vi "ArduinoCommand.vi"(8 "entrée d'erreur (pas d'erreur)":errorcluster, 10 "buffer à écrire":string, 11 "Refnum VISA en entrée":refnum<visa-resource-name>) -> (0 "sortie d'erreur":errorcluster, 2 "read buffer":string, 3 "Refnum VISA en sortie":refnum<visa-resource-name>)   [LabVIEW 2014, in "ShootingStar.lvlib"]
uses:
  ShootingStar.lvlib
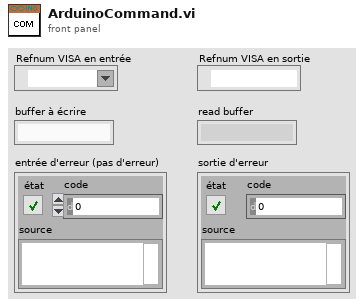
[diagram p1: front panel]
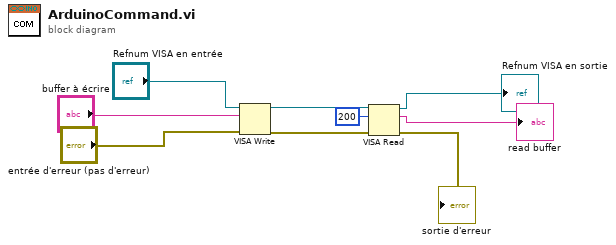
[diagram p0: block diagram]
diagram:
  n1 = VISA Write(VISA resource name="Refnum VISA en entrée", write buffer="buffer à écrire", error in (no error)="entrée d'erreur (pas d'erreur)") -> (VISA resource name out=w1:refnum<visa-resource-name>, error out=w2:errorcluster)  [unwired: 1 out]
  n2 = VISA Read(VISA resource name=w1, byte count=u32 200 ("nombre d'octets"), error in (no error)=w2) -> (VISA resource name out=→"Refnum VISA en sortie":refnum<visa-resource-name>, read buffer=→"read buffer":string, error out=→"sortie d'erreur":errorcluster)  [unwired: 1 out]
